vi "22.vi"(9 "2":dbl, 10 "Numeric":i32, 11 "Numeric 2":i32) -> (3 "Array":u32[](array[numeric]))   [LabVIEW 2016]
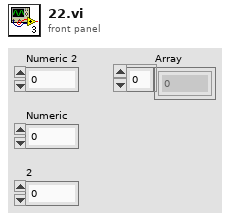
[diagram p1: front panel]
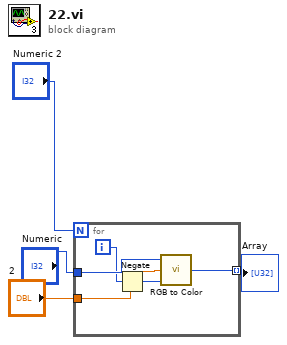
[diagram p0: block diagram]
diagram:
  n1 = for {
    N: "Numeric 2" -> [_]
    tunnel: [w9] -> w1 mode=indexing
    tunnel: "Numeric" -> [w7]
    tunnel: "2" -> [w8]
    i -> [w5]
    n2 = Negate(x=w5) -> (-x=w6:i32)
    n3 = call <vilib>:"RGB to Color.vi"("B"=w6, "G"=w8, "R"=w7) -> ("Color"=w9:u32)
  }
  "Array" <- w1
